vi "Periodic Tasks.vi"(8 "error in":errorcluster) -> ()   [LabVIEW 2019]
doc: "This VI runs in parallel to other tasks. It can contain as many user-defined periodic loops as you need. These can carry out PID or other sorts of timed response."
uses:
  <vilib>/Rock Robotics/WPI/DriverStation/WPI_DriverStationRobotMode2.ctl
  <vilib>/Rock Robotics/WPI/Utilities/WPI_GetSetVariantRefNum.vi
  Robot Global Data.vi
  <vilib>/Rock Robotics/Network Tables/NT Write Boolean.vi
  <vilib>/Rock Robotics/Network Tables/NT Write Number.vi
  <vilib>/Rock Robotics/Network Tables/NT Read Boolean.vi
  <vilib>/Rock Robotics/Network Tables/NT Read Number.vi
  <vilib>/Rock Robotics/WPI/RobotDrive/WPI_RobotDriveArcadeDrive_Standard(NoSaturation).vi
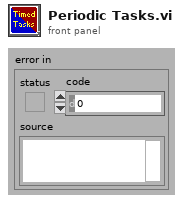
[diagram p1: front panel]
types:
  T1 = typedef "WPI_JoystickDevRef.ctl" = cluster{"Device":T2}
  T2 = typedef "WPI_JoystickDeviceEnum.ctl" = enum16{"USB 0", "USB 1", "USB 2", "USB 3", "USB 4", "USB 5"}
  T3 = typedef "WPI_RobotDriveDevRef.ctl" = cluster{"DevStatus":errorcluster, "Motors[]":T4[], "Square Inputs":bool, "Max Output":dbl}
  T4 = typedef "WPI_MotorControlDeviceRef.ctl" = cluster{"DeviceStatus":errorcluster, "Type":T5, "PWM":cluster{"PWM Channel":T6, "DeadBand":T7}, "CAN":cluster{"Device Number":u8, "SetOutput VI Ref":variant, "GetOutput VI Ref":variant, "Enable VI Ref":variant, "Disable VI Ref":variant, "Data":variant}, "Invert":bool, "DIO PWM":cluster{"PWM \"Enable\" Channel":T6, "DIOChannel":T8, "PWM Rate":dbl}}
  T5 = typedef "WPI_MotorControlType.ctl" = enum16{"PWM", "CAN", "DIO PWM"}
  T6 = typedef "FPGA_DIOPWMChannel.ctl" = enum8{"PWM 0", "PWM 1", "PWM 2", "PWM 3", "PWM 4", "PWM 5", "PWM 6", "PWM 7", "PWM 8", "PWM 9", "PWM MXP 0", "PWM MXP 1", "PWM MXP 2", "PWM MXP 3", "PWM MXP 4", "PWM MXP 5", "PWM MXP 6", "PWM MXP 7", "PWM MXP 8", "PWM MXP 9", "Invalid"}
  T7 = typedef "WPI_PWMDeadband.ctl" = cluster{"Name":string, "maxPositivePwm":i32, "minPositivePwm":i32, "centerPwm":i32, "maxNegativePwm":i32, "minNegativePwm":i32, "angularRange":u16}
  T8 = typedef "FPGA_DIOChannel.ctl" = enum8{"DIO 0", "DIO 1", "DIO 2", "DIO 3", "DIO 4", "DIO 5", "DIO 6", "DIO 7", "DIO 8", "DIO 9", "DIO MXP 0", "DIO MXP 1", "DIO MXP 2", "DIO MXP 3", "DIO MXP 4", "DIO MXP 5", "DIO MXP 6", "DIO MXP 7", "DIO MXP 8", "DIO MXP 9", "DIO MXP 10", "DIO MXP 11", "DIO MXP 12", "DIO MXP 13", "DIO MXP 14", "DIO MXP 15", "SPI Port CS1", "SPI Port CS2", "SPI Port CS3", "SPI Port MISO", "SPI Port MOSI", "Invalid"}
  T9 = cluster{"JoystickDevRef":T1, "RobotDriveDevRef":T3}
  T10 = typedef "WPI_DriverStationRobotMode2.ctl" = enum16{"Autonomous Disabled", "Autonomous Enabled", "Teleop Disabled", "Teleop Enabled", "Disconnected", "Finish", "Test Disabled", "Test Enabled", "Emergency Stopped"}
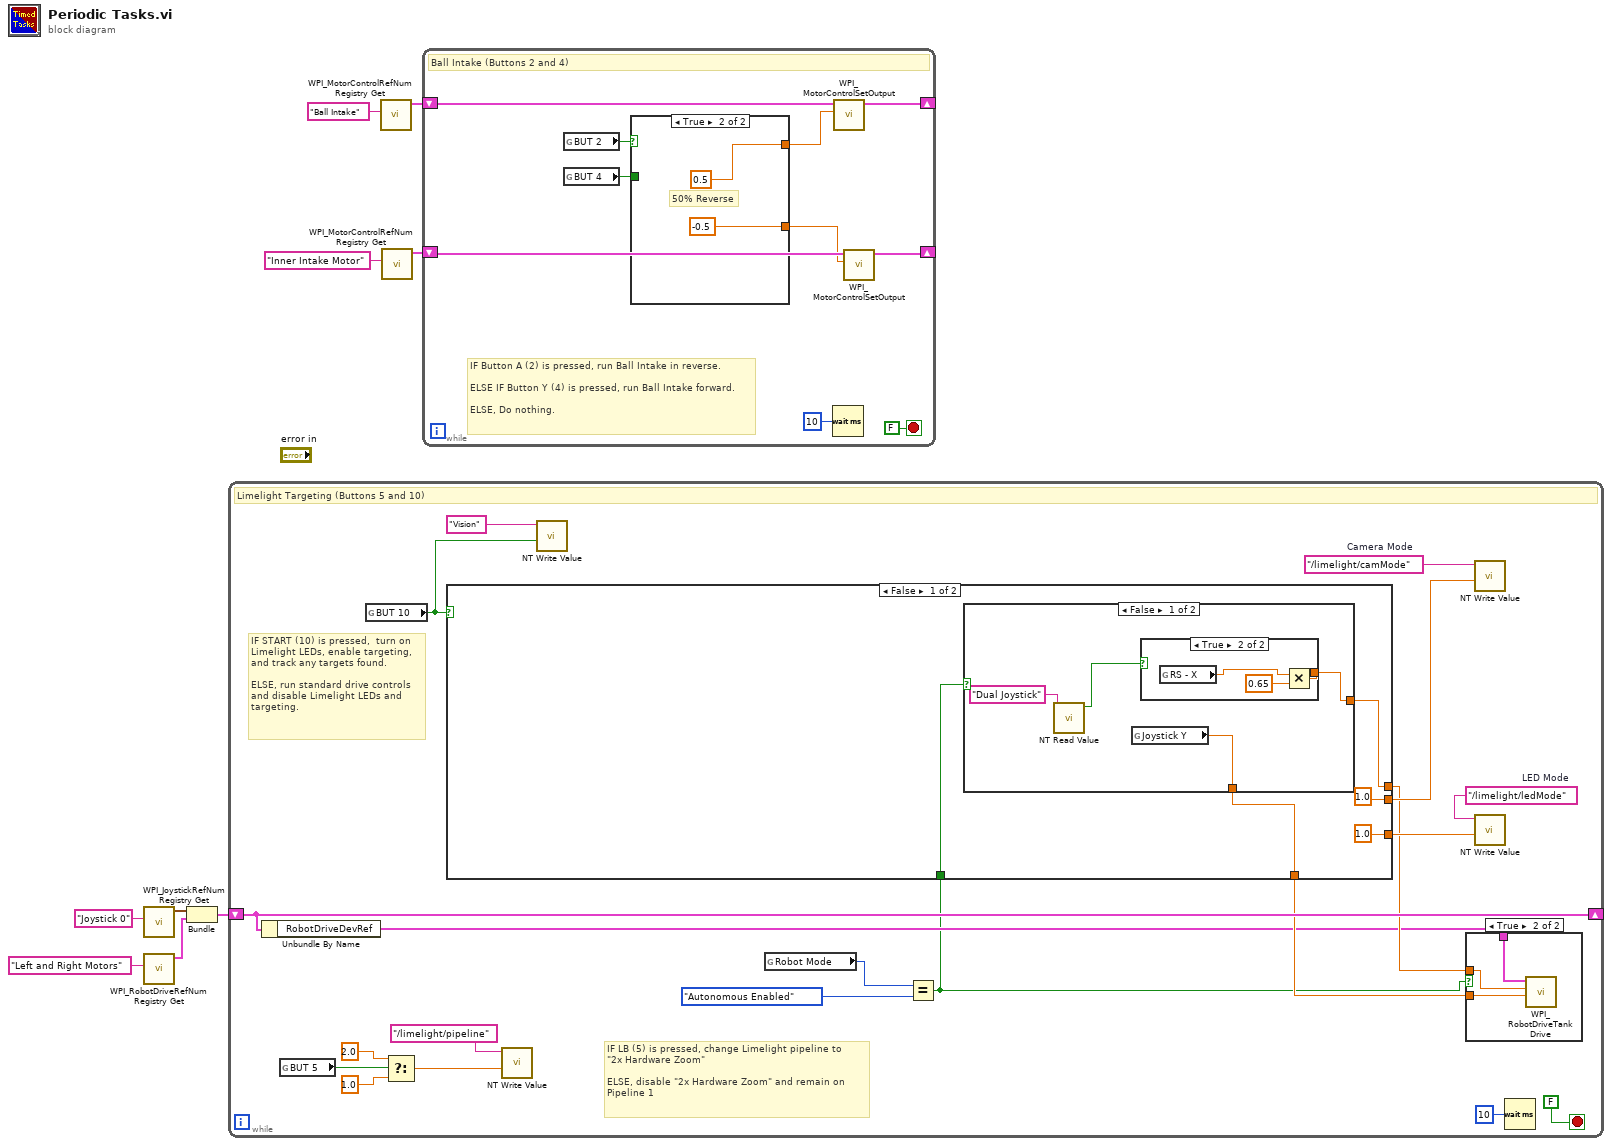
[diagram p0: block diagram]
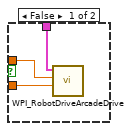
[diagram p2: hidden frame]
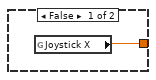
[diagram p3: hidden frame]
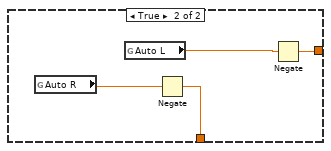
[diagram p4: hidden frame]
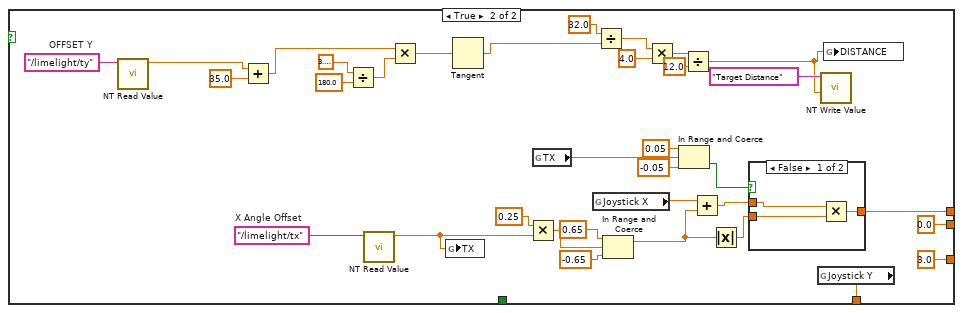
[diagram p5: hidden frame]
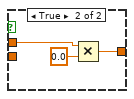
[diagram p6: hidden frame]
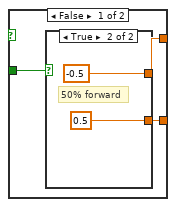
[diagram p7: hidden frame]
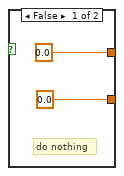
[diagram p8: hidden frame]
diagram:
  n1 = call <vilib>:"WPI_JoystickRefNum Registry Get.vi"("refnum name"="Joystick 0") -> ("JoystickDevRef"=w5:T1)  [unwired: 1 in, 9 out]
  n2 = call <vilib>:"WPI_RobotDriveRefNum Registry Get.vi"("refnum name"="Left and Right Motors") -> ("RobotDriveDevRef"=w4:T3)  [unwired: 1 in, 9 out]
  n3 = Bundle("JoystickDevRef"=w5, "RobotDriveDevRef"=w4) -> (w3:T9)  [unwired: 1 out]
  n4 = while {
    shift-right: [w28] -> _
    shift-left: w3 -> [w28]
    stop <- FALSE stop-if-true
    w26 = "/limelight/camMode"  # Camera Mode
    w27 = "/limelight/ledMode"  # LED Mode
    # "IF LB (5) is pressed, change Limelight pipeline to \n\"2x Hardware Zoom\"\n\nELSE, disable \"2x Hardware Zoom\" and remain on\nPipeline 1"
    # "IF START (10) is pressed,  turn on\nLimelight LEDs, enable targeting,\nand track any targets found.\n\nELSE, run standard drive controls\nand disable Limelight LEDs and \ntargeting."
    # "Limelight Targeting (Buttons 5 and 10)"
    n5 = Unbundle By Name(w28) -> ("RobotDriveDevRef"=w13:T3)
    n6 = global read "Robot Global Data.vi" "BUT 5"() -> (w16:bool)
    n7 = global read "Robot Global Data.vi" "BUT 10"() -> (w22:bool)
    n8 = Select(t=2.0, s=w16, f=1.0) -> (s? t:f=w19:dbl)
    n9 = call-poly <vilib>:"NT Write Value.vi"("Numeric"=w19, "Name"="/limelight/pipeline") -> ()  [unwired: 9 in, 1 out]
    n10 = call-poly <vilib>:"NT Write Value.vi"("Boolean"=w22, "Name"="Vision") -> ()  [unwired: 9 in, 1 out]
    n11 = global read "Robot Global Data.vi" "Robot Mode"() -> (w12:T10)
    n12 = Equal?(x=w12, y=WPI_DriverStationRobotMode2."Autonomous Enabled") -> (x = y?=w10:bool)
    n13 = case shown="False" w22 {
      tunnel: [1.0 ("Numeric") 0.0 ("Numeric")] -> w25
      tunnel: [1.0 ("Numeric") 3.0 ("Numeric")] -> w24
      tunnel: [w37 w79] -> w14
      tunnel: [w38 w78] -> w15
      tunnel: w10 -> [w36 _]
      frame False {
        n14 = case shown="False" w36 {
          tunnel: [w41 w50] -> w38
          tunnel: [w42 w52] -> w37
          frame False {
            n15 = call-poly <vilib>:"NT Read Value.vi"("Name"="Dual Joystick") -> ("Boolean"=w43:bool)  [unwired: 9 in, 1 out]
            n16 = global read "Robot Global Data.vi" "Joystick Y"() -> (w41:dbl)
            n17 = case shown="True" w43 {
              tunnel: [w45 w46] -> w42
              frame False {
                n18 = global read "Robot Global Data.vi" "Joystick X"() -> (w45:dbl)
              }
              frame True {
                n19 = global read "Robot Global Data.vi" "RS - X"() -> (w47:dbl)
                n20 = Multiply(x=w47, y=0.65) -> (x*y=w46:dbl)
              }
            }
          }
          frame True {
            n21 = global read "Robot Global Data.vi" "Auto R"() -> (w49:dbl)
            n22 = global read "Robot Global Data.vi" "Auto L"() -> (w51:dbl)
            n23 = Negate(x=w49) -> (-x=w50:dbl)
            n24 = Negate(x=w51) -> (-x=w52:dbl)
          }
        }
      }
      frame True {
        w62 = "/limelight/ty"  # OFFSET Y
        w80 = "/limelight/tx"  # X Angle Offset
        n25 = call-poly <vilib>:"NT Read Value.vi"("Name"=w62) -> ("Numeric"=w60:dbl)  [unwired: 9 in, 1 out]
        n26 = Add(x=w60, y=35.0) -> (x+y=w58:dbl)
        n27 = Divide(x=3.141592653589793, y=180.0) -> (x/y=w68:dbl)
        n28 = call-poly <vilib>:"NT Read Value.vi"("Name"=w80) -> ("Numeric"=w84:dbl)  [unwired: 9 in, 1 out]
        n29 = Multiply(x=w58, y=w68) -> (x*y=w67:dbl)
        n30 = global write "Robot Global Data.vi" "TX"(w84) -> ()
        n31 = Tangent(1:w67) -> (0:w66:dbl)
        n32 = Multiply(x=0.25 ("y"), y=w84) -> (x*y=w81:dbl)
        n33 = global read "Robot Global Data.vi" "TX"() -> (w74:dbl)
        n34 = global read "Robot Global Data.vi" "Joystick X"() -> (w72:dbl)
        n35 = Divide(x=32.0, y=w66) -> (x/y=w57:dbl)
        n36 = In Range and Coerce(upper limit=0.65, x=w81, lower limit=-0.65) -> (coerced(x)=w69:dbl)  [unwired: 1 out]
        n37 = Multiply(x=w57, y=4.0) -> (x*y=w55:dbl)
        n38 = In Range and Coerce(upper limit=0.05, x=w74, lower limit=-0.05) -> (In Range?=w77:bool)  [unwired: 1 out]
        n39 = Divide(x=w55, y=12.0) -> (x/y=w53:dbl)
        n40 = Add(x=w72, y=w69) -> (x+y=w71:dbl)
        n41 = Absolute Value(x=w69) -> (abs(x)=w70:dbl)
        n42 = case shown="False" w77 {
          tunnel: [w89 w91] -> w79
          tunnel: w71 -> [w88 w90]
          tunnel: w70 -> [w87 _]
          frame False {
            n43 = Multiply(x=w88, y=w87) -> (x*y=w89:dbl)
          }
          frame True {
            n44 = Multiply(x=w90, y=0.0) -> (x*y=w91:dbl)
          }
        }
        n45 = global read "Robot Global Data.vi" "Joystick Y"() -> (w78:dbl)
        n46 = call-poly <vilib>:"NT Write Value.vi"("Numeric"=w53, "Name"="Target Distance") -> ()  [unwired: 9 in, 1 out]
        n47 = global write "Robot Global Data.vi" "DISTANCE"(w53) -> ()
      }
    }
    n48 = case shown="True" w10 {
      tunnel: w15 -> [w32 w33]
      tunnel: w14 -> [w31 w34]
      tunnel: w13 -> [w30 w35]
      frame False {
        n49 = call-poly <vilib>:"WPI_RobotDriveArcadeDrive.vi"("Y axis value"=w32, "X axis value"=w31, "RobotDriveDevRef"=w30) -> ()  [unwired: 6 in, 3 out]
      }
      frame True {
        n50 = call <vilib>:"WPI_RobotDriveTankDrive.vi"("Right axis value"=w33, "Left axis value"=w34, "RobotDriveDevRef"=w35) -> ()  [unwired: 6 in, 3 out]
      }
    }
    n51 = call-poly <vilib>:"NT Write Value.vi"("Numeric"=w25, "Name"=w26) -> ()  [unwired: 9 in, 1 out]
    n52 = call-poly <vilib>:"NT Write Value.vi"("Numeric"=w24, "Name"=w27) -> ()  [unwired: 9 in, 1 out]
    n53 = Wait (ms)(milliseconds to wait=u32 10) -> ()  [unwired: 1 out]
  }
  n54 = call <vilib>:"WPI_MotorControlRefNum Registry Get.vi"("refnum name"="Ball Intake") -> ("MotorControlDevRef"=w9:T4)  [unwired: 9 in, 1 out]
  n55 = call <vilib>:"WPI_MotorControlRefNum Registry Get.vi"("refnum name"="Inner Intake Motor") -> ("MotorControlDevRef"=w1:T4)  [unwired: 9 in, 1 out]
  n56 = while {
    shift-right: [w99] -> _
    shift-left: w9 -> [w98]
    shift-right: [w95] -> _
    shift-left: w1 -> [w94]
    stop <- FALSE stop-if-true
    # "IF Button A (2) is pressed, run Ball Intake in reverse. \n\nELSE IF Button Y (4) is pressed, run Ball Intake forward.\n\nELSE, Do nothing."
    # "Ball Intake (Buttons 2 and 4)"
    n57 = global read "Robot Global Data.vi" "BUT 2"() -> (w101:bool)
    n58 = global read "Robot Global Data.vi" "BUT 4"() -> (w102:bool)
    n59 = case shown="True" w101 {
      tunnel: [w105 0.5 ("Output")] -> w100
      tunnel: w102 -> [w104 _]
      tunnel: [w103 -0.5 ("Output")] -> w93
      frame False {
        n60 = case shown="True" w104 {
          tunnel: [0.0 ("Output") -0.5 ("Output")] -> w105
          tunnel: [0.0 ("Output") 0.5 ("Output")] -> w103
          frame False {
            # "do nothing"
          }
          frame True {
            # "50% forward"
          }
        }
      }
      frame True {
        # "50% Reverse"
      }
    }
    n61 = Wait (ms)(milliseconds to wait=u32 10) -> ()  [unwired: 1 out]
    n62 = call <vilib>:"WPI_MotorControlSetOutput.vi"("Output"=w100, "MotorControlDevRef"=w98) -> ("MotorControlDevRef"=w99:T4)  [unwired: 7 in, 2 out]
    n63 = call <vilib>:"WPI_MotorControlSetOutput.vi"("Output"=w93, "MotorControlDevRef"=w94) -> ("MotorControlDevRef"=w95:T4)  [unwired: 7 in, 2 out]
  }
